vi "S2DS_Initialization (SubVI).vi"(9 "False channel":string[][](array[string]), 10 "User info":string[](array[string]), 11 "All channel parameters (in)":T3 {"Scan parameters"."Y data taking" items=["in both direction", "in up direction only", "in down direction only"]; "Scan parameters"."X data taking" items=["in both direction", "in up direction only", "in down direction only"]}) -> (1 "Data save info (out)":T1={"File path"=path "", "Header"="", "File name"="", "False channel"=[], "Channel names"=[], "Buffer size"=0, "Format"="%.6f"}, 2 "All channel info (out)":T2, 3 "All channel parameters (out)":T3 {"Scan parameters"."Y data taking" items=["in both direction", "in up direction only", "in down direction only"]; "Scan parameters"."X data taking" items=["in both direction", "in up direction only", "in down direction only"]})   [LabVIEW 2025]
uses:
  TYPE DEFS/S2DS_All Channel Parameters.ctl
  TYPE DEFS/S2DS_WC info.ctl
  TYPE DEFS/S2DS_Single WC info.ctl
  TYPE DEFS/S2DS_RC info.ctl
  TYPE DEFS/S2DS_Single RC info.ctl
  TYPE DEFS/S2DS_DAC info new.ctl
  TYPE DEFS/S2DS_Single DC info.ctl
  TYPE DEFS/S2DS_Array Inst Info.ctl
  TYPE DEFS/S2DS_Sweep Info.ctl
  TYPE DEFS/S2DS_Display info.ctl
  TYPE DEFS/S2DS_Data saving info.ctl
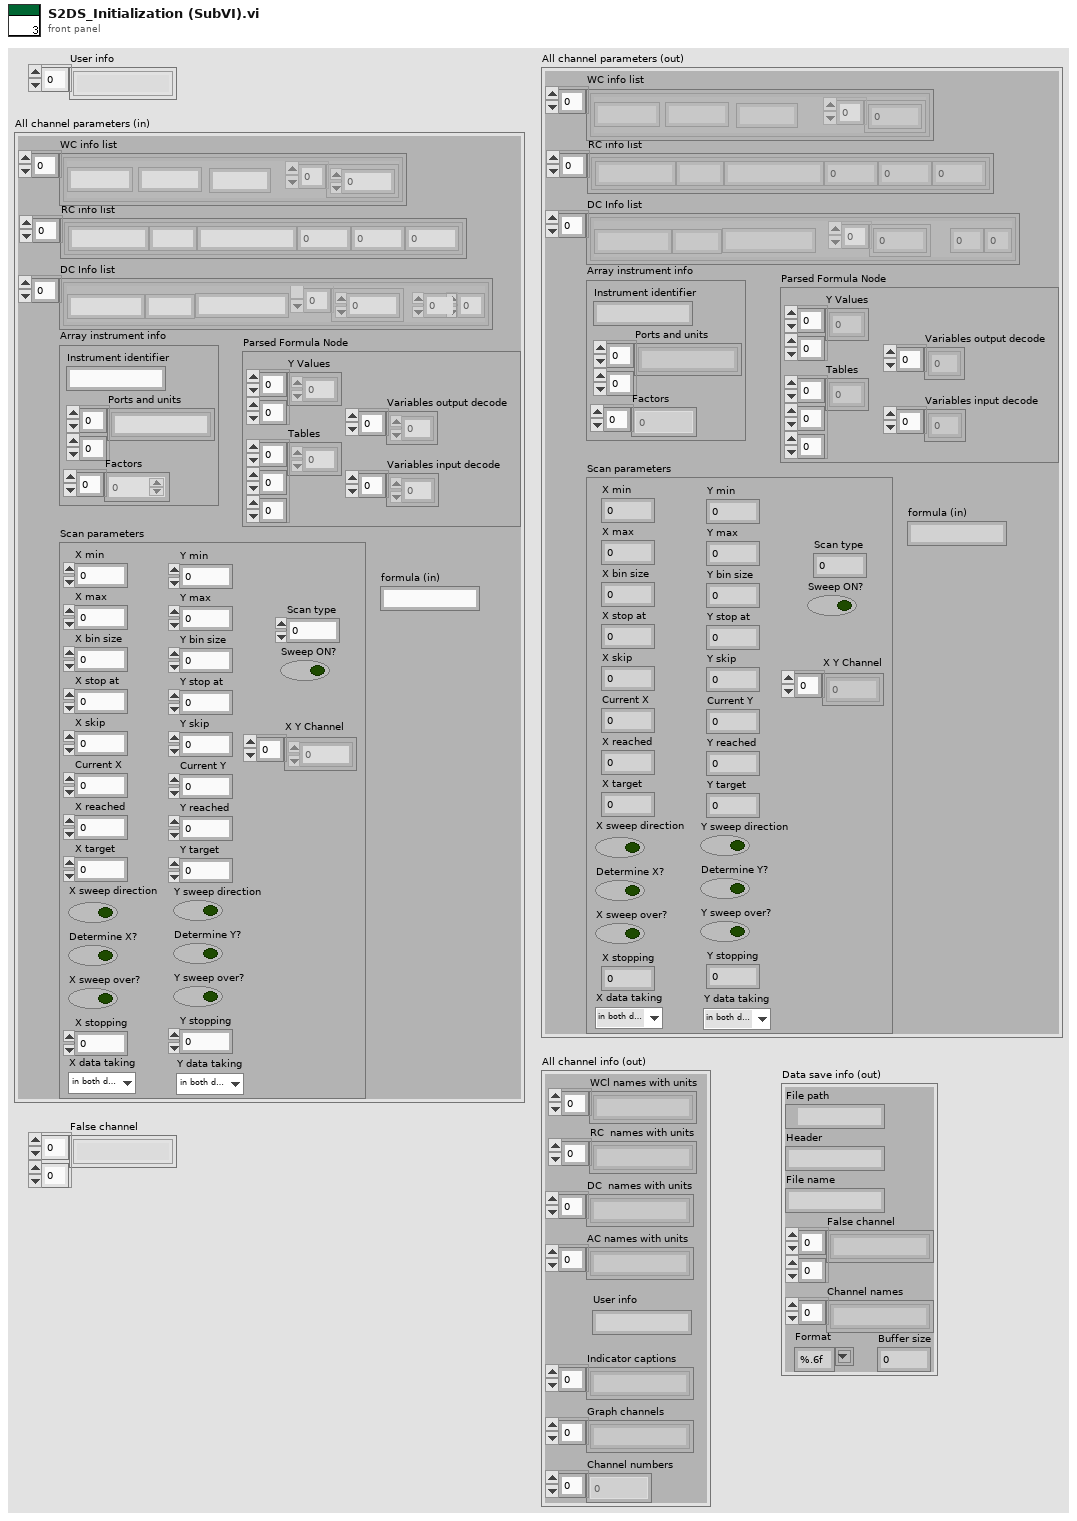
[diagram p1: front panel]
types:
  T1 = typedef "S2DS_Data saving info.ctl" = cluster{"File path":path, "Header":string, "File name":string, "False channel":string[][], "Channel names":string[], "Buffer size":i32, "Format":string}
  T2 = typedef "S2DS_Display info.ctl" = cluster{"WCl names with units":string[], "RC  names with units":string[], "DC  names with units":string[], "AC names with units":string[], "Indicator captions":string[], "Graph channels":string[], "Channel numbers":i32[], "User info":string}
  T3 = typedef "S2DS_All Channel Parameters.ctl" = cluster{"WC info list":T4, "RC info list":T6, "DC Info list":T8, "Array instrument info":T10, "Scan parameters":T11, "Parsed Formula Node":cluster{"Y Values":dbl[][], "Tables":i32[][][], "Variables input decode":i32[], "Variables output decode":i32[]}, "formula (in)":string}
  T4 = typedef "S2DS_WC info.ctl" = T5[]
  T5 = typedef "S2DS_Single WC info.ctl" = cluster{"Instrument identifier":string, "Write channel parameters":dbl[], "Name":string, "Unit":string}
  T6 = typedef "S2DS_RC info.ctl" = T7[]
  T7 = typedef "S2DS_Single RC info.ctl" = cluster{"Instrument identifier":string, "Factor":dbl, "Averaging":i32, "Wait (ms)":i32, "Unit":string, "Name":string}
  T8 = typedef "S2DS_DAC info new.ctl" = T9[]
  T9 = typedef "S2DS_Single DC info.ctl" = cluster{"Operation identifier":string, "DC parameters":dbl[], "U":i32, "V":i32, "Name":string, "Unit":string}
  T10 = typedef "S2DS_Array Inst Info.ctl" = cluster{"Instrument identifier":string, "Ports and units":string[][], "Factors":dbl[]}
  T11 = typedef "S2DS_Sweep Info.ctl" = cluster{"X min":ext, "X max":dbl, "Y min":dbl, "Y max":dbl, "X bin size":dbl, "Y bin size":dbl, "X stop at":dbl, "Y stop at":dbl, "X skip":u64, "Y skip":u64, "Current X":dbl, "Current Y":dbl, "X reached":i32, "Y reached":i32, "X target":dbl, "Y target":dbl, "Sweep ON?":bool, "X sweep direction":bool, "Y sweep direction":bool, "Determine X?":bool, "Determine Y?":bool, "X sweep over?":bool, "Y sweep over?":bool, "Scan type":i32, "X stopping":i32, "Y stopping":i32, "X Y Channel":u16[], "X data taking":u16, "Y data taking":u16}
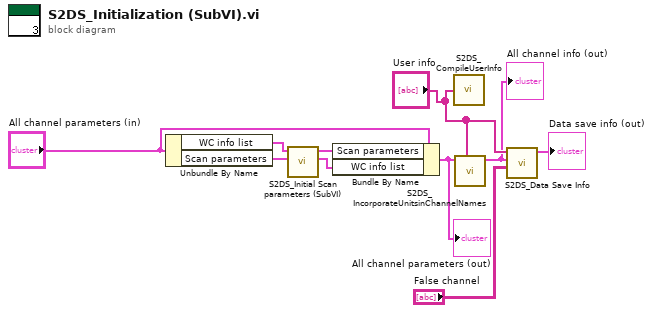
[diagram p0: block diagram]
diagram:
  n1 = Unbundle By Name("All channel parameters (in)") -> ("WC info list"=w10:T4, "Scan parameters"=w2:T11)
  n2 = call "S2DS_Initial Scan parameters (SubVI).vi"("Scan parameters (in)"=w2, "WC info list"=w10) -> ("WC Info list out"=w1:T5[], "Scan parameters out"=w6:T11)  [unwired: 8 in]
  n3 = Bundle By Name(cluster="All channel parameters (in)", "Scan parameters"=w6, "WC info list"=w1) -> (w9:T3)
  "All channel parameters (out)" <- w9
  n4 = call "S2DS_CompileUserInfo.vi"("User info"="User info") -> ()  [unwired: 1 out]
  n5 = call "S2DS_IncorporateUnitsinChannelNames.vi"("User info"="User info", "All channel parameters (in)"=w9) -> ("All channel info (out)"=w5:T2)  [unwired: 7 in]
  "All channel info (out)" <- w5
  n6 = call "S2DS_Data Save Info.vi"("User info"="User info", "All channel info (in)"=w5, "False channels"="False channel") -> ("Data save info (out)"=→"Data save info (out)":T1)  [unwired: 7 in]
